vi "BKTest.vi"() -> ()   [LabVIEW 2021]
panel:
  out "BK Impedance Measurement":string
  in  "VISA resource name":refnum<visa-resource-name>
  # "Change the range by double\n clicking the max value on the scale"
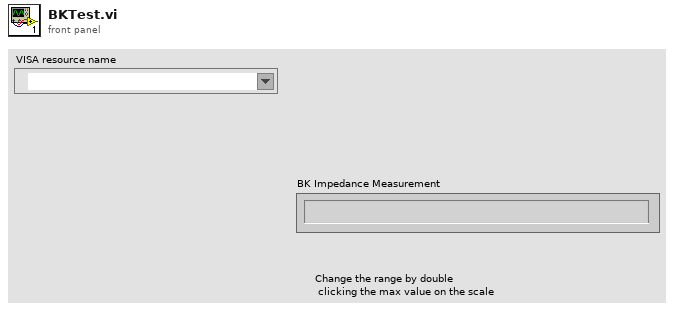
[diagram p1: front panel]
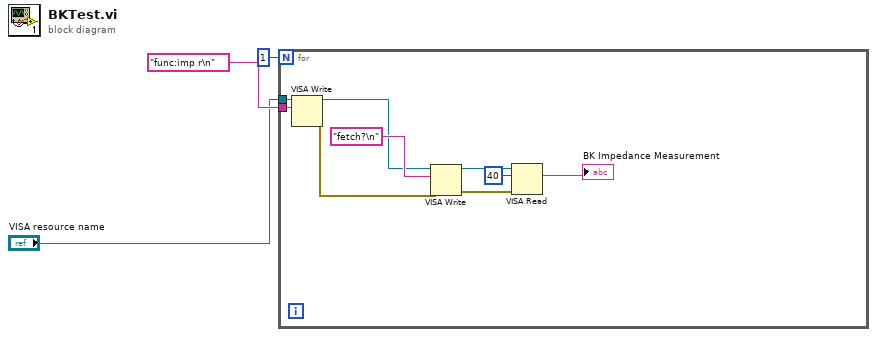
[diagram p0: block diagram]
diagram:
  n1 = for {
    N: 1 -> [_]
    tunnel: "func:imp r\n" ("write buffer") -> [w12]
    tunnel: "VISA resource name" -> [w11]
    n2 = VISA Write(VISA resource name=w11, write buffer=w12) -> (VISA resource name out=w5:refnum<visa-resource-name>, error out=w6:errorcluster)  [unwired: 1 in, 1 out]
    n3 = VISA Write(VISA resource name=w5, write buffer="fetch?\n", error in (no error)=w6) -> (VISA resource name out=w9:refnum<visa-resource-name>, error out=w8:errorcluster)  [unwired: 1 out]
    n4 = VISA Read(VISA resource name=w9, byte count=u32 40, error in (no error)=w8) -> (read buffer=→"BK Impedance Measurement":string)  [unwired: 3 out]
  }
